vi "ErrorHandler.vi"(8 "error in (no error)":errorcluster, 11 "Master State in":T1) -> (0 "error out":errorcluster, 3 "Master State out":T1)   [LabVIEW 2019]
uses:
  Typedefs/#enum_MasterState.ctl
  LowLevelError.vi
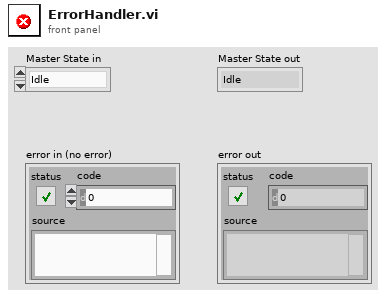
[diagram p1: front panel]
types:
  T1 = typedef "#enum_MasterState.ctl" = enum16{"Idle", "Init", "Close", "Error"}
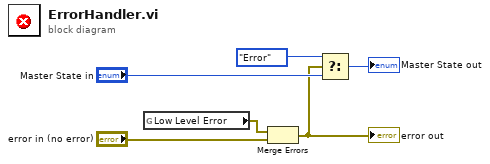
[diagram p0: block diagram]
diagram:
  n1 = global read "LowLevelError.vi" "Low Level Error"() -> (w1:errorcluster)
  n2 = Merge Errors(w1, "error in (no error)") -> (w3:errorcluster)
  "error out" <- w3
  n3 = Select(t=#enum_MasterState."Error", s=w3, f="Master State in") -> (s? t:f=→"Master State out":T1)
